vi "Klinger Goto.vi"(0 "Axe":u8(ring) items=["W", "X", "Y", "Z"], 1 "Suivi":T1={"CorrectPos"=TRUE, "Nb Essais Max"=5, "Erreur de suivi max"=1.0}, 2 "Moving Ref":refnum<vi>, 5 "Relatif":bool caption="Relatif/Absolu\n(Absolu)", 7 "UnitDem":u8(ring)=2 caption="Unités" items=["Pas", "mm", "ps"], 9 "PosDem":dbl=1.0 caption="Allez à" min=-7999999.9 max=7999999.9 step=0.1 format="%#_8f", 11 "error in":errorcluster, 12 "Position Ref":refnum<vi>) -> (3 "Moving":bool caption="Déplacement\nen cours", 4 "PLimit":bool caption="Limite +", 6 "NLimit":bool caption="Limite -", 8 "Pos Init":dbl caption="Position Initiale", 10 "Position":dbl format="%#.1f", 13 "PosErreur":dbl caption="Erreur de\nPositionnement", 14 "Indcomm":string caption="Indicateur de commande", 15 "error out":errorcluster)   [LabVIEW 2010]
doc: "Ce VI envoie une commande de déplacement au controlleur Klinger MC4. \n\nAxe : Sélectionner l'axe sur lequel effectuer le déplacement\n\nAllez à :En mode de déplacement absolu, entrer la position de destination en pas. En mode de déplacement relatif, entrer le nombre de pas à effectuer. Le signe indique la direcetion de déplacement. Valeur accepter :-7 999 999,9 à 7 999 999,9\n\nRelatif/Absolu : Choisi le type de déplacementà effectuer. En mode absolu, le déplacement est effectué par rapport à une position de référence prédéfini. En mode relatif, le déplacement est effectué par rapport à la position actuelle.\n\nLimite + : Indique l'atteinte de l'interrupeur de fin de course positif\n\nLimite - : Indique l'atteinte de l'interrupeur de fin de course négatif\n\nPosition: Indique la position finale"
uses:
  <vilib>/Utility/error.llb/DialogType.ctl
  Programmes LabView/Réflectivité Différentielle/Params Globals.vi
  <userlib>/Klinger/Klinger Lib.llb/Klinger ConvUnitSgl.vi
panel:
  out "NbEssais":i32
  out "Message D'erreur":string
  out "Erreur":bool
  # "Relatif"
  # "Absolu"
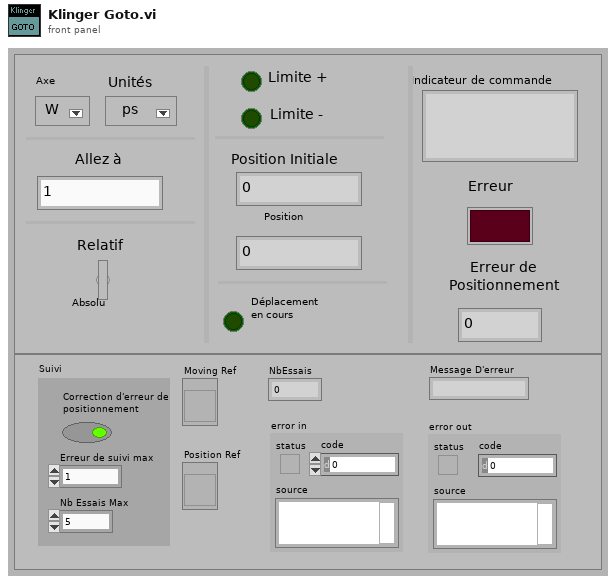
[diagram p1: front panel]
types:
  T1 = cluster{"CorrectPos":bool, "Nb Essais Max":i32, "Erreur de suivi max":dbl}
  T2 = enum16{"Dem Pos Init", "Lire Pos Init", "Envoie Comm", "Dem Statut", "Lire Statut", "Attend RQS", "Erreur GPIB", "Dépl incomp", "Dépl comp"}
  T3 = typedef "DialogType.ctl" = u16
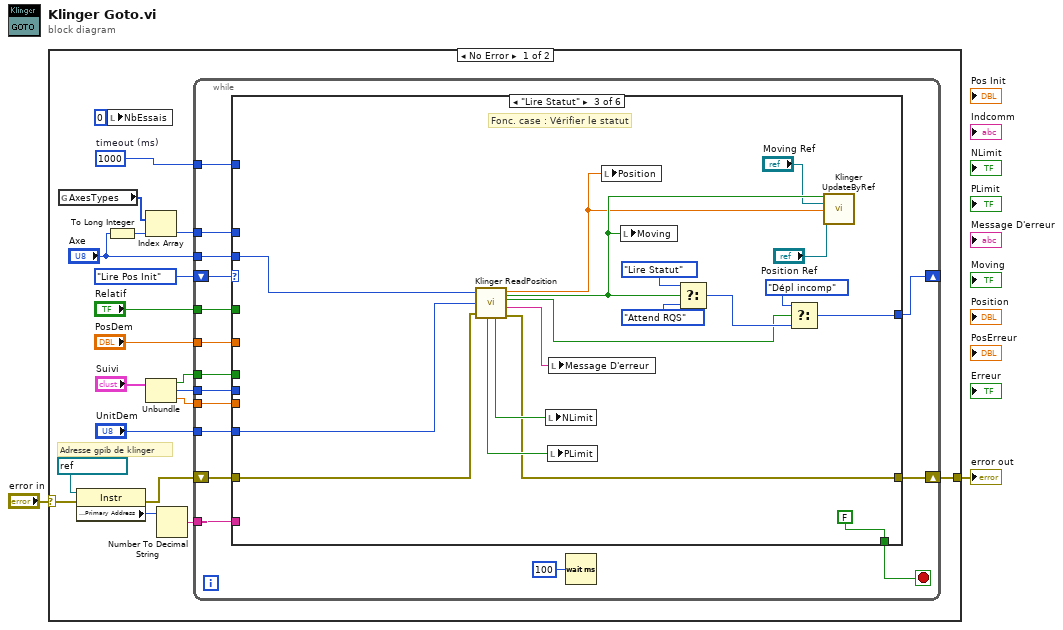
[diagram p0: block diagram]
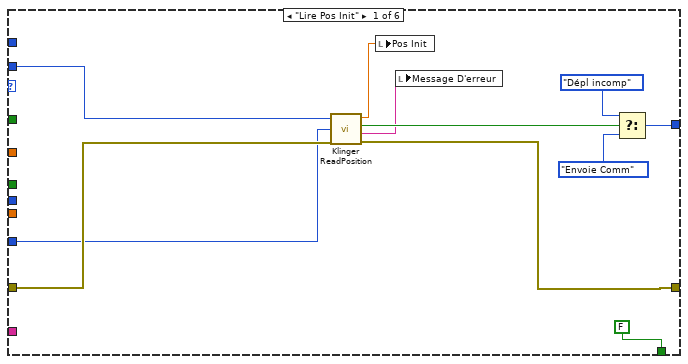
[diagram p2: hidden frame]
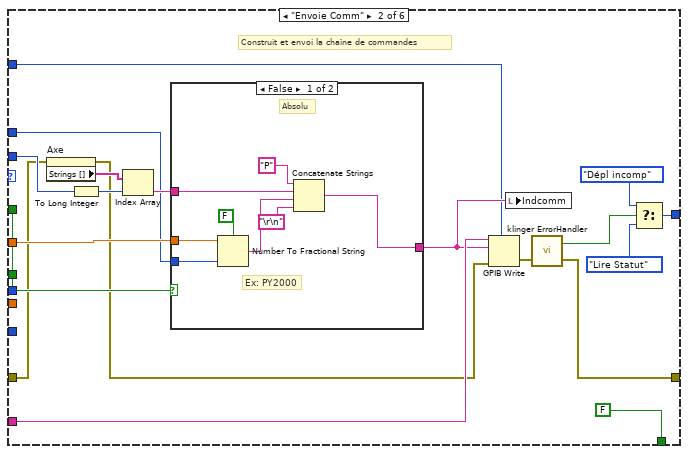
[diagram p3: hidden frame]
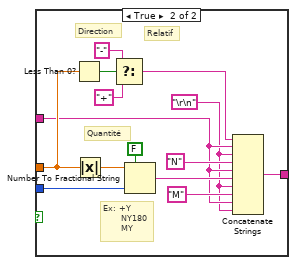
[diagram p4: hidden frame]
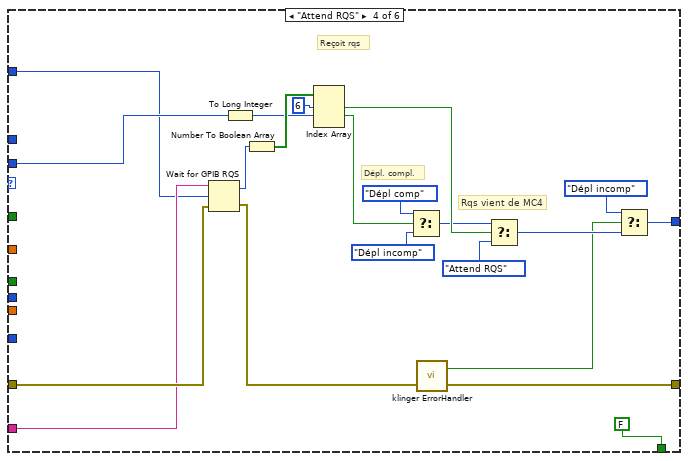
[diagram p5: hidden frame]
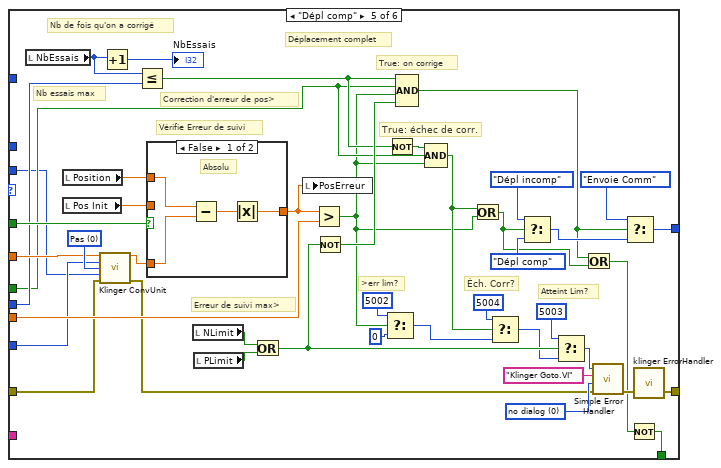
[diagram p6: hidden frame]
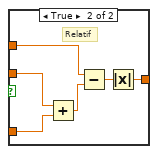
[diagram p7: hidden frame]
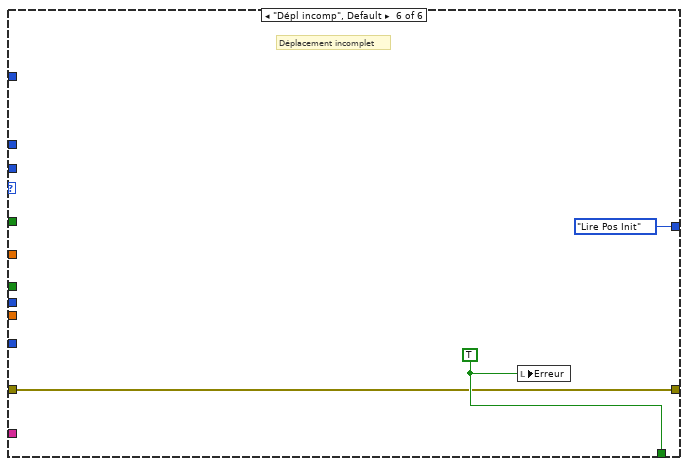
[diagram p8: hidden frame]
diagram:
  n1 = case shown="No Error" "error in" {
    selector: "error in" -> [w15 w187]
    tunnel: [w20 w187] -> w2
    frame No Error {
      w12 = 1000  # timeout (ms)
      # "Adresse gpib de klinger"
      n2 = global read "Params Globals.vi" "AxesTypes"() -> (w3:enum16{"UE30", "UE72"}[])
      n3 = property class="Instr"(reference=refnum<visa-resource-name> "KLINGER", error in=w15) -> (error out=w14:errorcluster, "GPIB Settings:Primary Address"=w18:u16)  [unwired: 1 out]
      n4 = To Long Integer(number="Axe") -> (32bit integer=w6:i32)
      n5 = local write "NbEssais"(0 ("Numeric")) -> ()
      n6 = Index Array(array=w3, index=w6) -> (element=w4:enum16{"UE30", "UE72"})
      n7 = Unbundle("Suivi") -> ("CorrectPos"=w8:bool, "Nb Essais Max"=w9:i32, "Erreur de suivi max"=w7:dbl)
      n8 = Number To Decimal String(number=w18) -> (decimal integer string=w16:string)  [unwired: 1 in]
      n9 = while {
        shift-right: [w37] -> w20
        shift-left: w14 -> [w36]
        tunnel: "Axe" -> [w35]
        tunnel: "PosDem" -> [w34]
        tunnel: "Relatif" -> [w33]
        tunnel: w12 -> [w32]
        shift-right: [w29] -> _
        shift-left: T2."Lire Pos Init" ("f") -> [w30]
        tunnel: w7 -> [w28]
        tunnel: w16 -> [w27]
        tunnel: "UnitDem" -> [w26]
        tunnel: w9 -> [w25]
        tunnel: w8 -> [w24]
        tunnel: w4 -> [w23]
        stop <- w38 stop-if-true
        n10 = case shown="\"Lire Statut\"" w30 {
          tunnel: [FALSE FALSE FALSE FALSE w166 w185] -> w38
          tunnel: [w45 w56 w95 w110 w163 w184] -> w37
          tunnel: w36 -> [w42 w52 w100 w129 w132 w184]
          tunnel: w35 -> [w41 w65 w91 w127 w133 _]
          tunnel: w34 -> [_ w54 _ _ w150 _]
          tunnel: w33 -> [_ w63 _ _ w173 _]
          tunnel: w27 -> [_ w62 _ w128 _ _]
          tunnel: w32 -> [_ w53 _ w118 _ _]
          tunnel: [w46 w59 w105 w113 w151 T2."Lire Pos Init" ("f")] -> w29
          tunnel: w28 -> [_ _ _ _ w172 _]
          tunnel: w26 -> [w39 _ w92 _ w149 _]
          tunnel: w25 -> [_ _ _ _ w135 _]
          tunnel: w24 -> [_ _ _ _ w134 _]
          tunnel: w23 -> [_ w50 _ _ _ _]
          frame "Lire Pos Init" {
            n11 = call <userlib>:"Klinger ReadPosition.vi"("Axe"=w41, "UnitDem"=w39, "error in"=w42) -> ("Position"=w40:dbl, "Statut"=w44:bool, "Cont Error"=w43:string, "error out"=w45:errorcluster)  [unwired: 1 in, 3 out]
            n12 = local write "Pos Init"(w40) -> ()
            n13 = local write "Message D'erreur"(w43) -> ()
            n14 = Select(t=T2."Dépl incomp", s=w44, f=T2."Envoie Comm") -> (s? t:f=w46:T2)
          }
          frame "Envoie Comm" {
            # "Construit et envoi la chaîne de commandes"
            n15 = property on="Axe" class="Ring (strict)"(error in=w52) -> (error out=w51:errorcluster, "Strings []"=w68:string[])  [unwired: 1 in, 1 out]
            n16 = To Long Integer(number=w65) -> (32bit integer=w64:i32)
            n17 = Index Array(array=w68, index=w64) -> (element=w67:string)
            n18 = case shown="False" w63 {
              tunnel: w54 -> [w76 w88]
              tunnel: w67 -> [w73 w80]
              tunnel: [w71 w78] -> w58
              tunnel: w50 -> [w69 w77]
              frame False {
                # "Ex: PY2000"
                # "Absolu"
                n19 = Number To Fractional String(use system decimal point (T)=FALSE, number=w76, precision (6)=w69) -> (F-format string=w75:string)  [unwired: 1 in]
                n20 = Concatenate Strings("P", w73, w75, "\r\n") -> (w71:string)
              }
              frame True {
                w79 = "\r\n"
                # "Quantité"
                # "Direction"
                # "Ex: +Y\n      NY180\n      MY"
                # "Relatif"
                n21 = Less Than 0?(x=w88) -> (x < 0?=w87:bool)
                n22 = Absolute Value(x=w88) -> (abs(x)=w90:dbl)
                n23 = Select(t="-", s=w87, f="+") -> (s? t:f=w84:string)
                n24 = Number To Fractional String(use system decimal point (T)=FALSE, number=w90, precision (6)=w77) -> (F-format string=w82:string)  [unwired: 1 in]
                n25 = Concatenate Strings(w84, w80, w79, "N", w80, w82, w79, "M", w80, w79) -> (w78:string)
              }
            }
            n26 = GPIB Write(0:w62, 1:w58, 3:w51, 4:w53) -> (6:w57:errorcluster)  [unwired: 1 in, 1 out]
            n27 = local write "Indcomm"(w58) -> ()
            n28 = call <userlib>:"klinger ErrorHandler.vi"("error in (no error)"=w57) -> ("error out"=w56:errorcluster, "Erreur"=w55:bool)  [unwired: 1 in]
            n29 = Select(t=T2."Dépl incomp", s=w55, f=T2."Lire Statut") -> (s? t:f=w59:T2)
          }
          frame "Lire Statut" {
            # "Fonc. case : Vérifier le statut"
            n30 = call <userlib>:"Klinger ReadPosition.vi"("Axe"=w91, "UnitDem"=w92, "error in"=w100) -> ("PLimit"=w99:bool, "Moving"=w96:bool, "Position"=w94:dbl, "Statut"=w101:bool, "NLimit"=w98:bool, "Cont Error"=w97:string, "error out"=w95:errorcluster)  [unwired: 1 in]
            n31 = local write "NLimit"(w98) -> ()
            n32 = local write "PLimit"(w99) -> ()
            n33 = local write "Message D'erreur"(w97) -> ()
            n34 = local write "Position"(w94) -> ()
            n35 = local write "Moving"(w96) -> ()
            n36 = Select(t=T2."Lire Statut", s=w96, f=T2."Attend RQS") -> (s? t:f=w103:T2)
            n37 = Select(t=T2."Dépl incomp", s=w101, f=w103) -> (s? t:f=w105:T2)
            n38 = call <userlib>:"Klinger UpdateByRef.vi"("Moving?"=w96, "Moving Ref"="Moving Ref", "Position"=w94, "Position Ref"="Position Ref") -> ()  [unwired: 11 in, 1 out]
          }
          frame "Attend RQS" {
            # "Dépl. compl."
            # "Rqs vient de MC4"
            # "Reçoit rqs"
            n39 = Wait for GPIB RQS(2:w129, 3:w118, 4:w128) -> (0:w117:errorcluster, 1:w125:i16)
            n40 = To Long Integer(number=w127) -> (32bit integer=w121:i32)
            n41 = Number To Boolean Array(number=w125) -> (Boolean array=w126:bool[])
            n42 = Index Array(array=w126, index #1=6 ("index"), index #2=w121) -> (element #1=w123:bool, element #2=w120:bool)  [unwired: 1 in, 1 out]
            n43 = Select(t=T2."Dépl comp", s=w120, f=T2."Dépl incomp") -> (s? t:f=w119:T2)
            n44 = call <userlib>:"klinger ErrorHandler.vi"("error in (no error)"=w117) -> ("error out"=w110:errorcluster, "Erreur"=w109:bool)  [unwired: 1 in]
            n45 = Select(t=w119, s=w123, f=T2."Attend RQS") -> (s? t:f=w112:T2)
            n46 = Select(t=T2."Dépl incomp", s=w109, f=w112) -> (s? t:f=w113:T2)
          }
          frame "Dépl comp" {
            w160 = u8 0 items=["Pas", "mm", "ps"] ("UnitAct")
            w168 = T3 0 items=["no dialog", "OK message", "continue or stop message", "OK message + warnings", "continue/stop + warnings"] ("type of dialog (OK msg:1)")
            # "Nb essais max"
            # "Correction d'erreur de pos>"
            # "Erreur de suivi max>"
            # ">err lim?"
            # "Éch. Corr?"
            # "Atteint Lim?"
            # "Nb de fois qu'on a corrigé"
            # "True: échec de corr."
            # "True: on corrige"
            # "Vérifie Erreur de suivi"
            # "Déplacement complet"
            n47 = local read "NbEssais"() -> (w158:i32)
            n48 = local read "Position"() -> (w164:dbl)
            n49 = local read "Pos Init"() -> (w165:dbl)
            n50 = call-poly <userlib>:"Klinger ConvUnit.vi"("ParamAct"=w150, "UnitDem"=w149, "UnitAct"=w160, "Axe"=w133, "error in"=w132) -> ("ParamDem"=w159:dbl, "error out"=w131:errorcluster)  [unwired: 9 in]
            n51 = Increment(x=w158) -> (x+1=→"NbEssais":i32)
            n52 = Less Or Equal?(x=w158, y=w135) -> (x <= y?=w153:bool)
            n53 = case shown="False" w173 {
              tunnel: w165 -> [_ w182]
              tunnel: w159 -> [w176 w181]
              tunnel: [w175 w179] -> w157
              tunnel: w164 -> [w174 w178]
              frame False {
                # "Absolu"
                n54 = Subtract(x=w174, y=w176) -> (x-y=w177:dbl)
                n55 = Absolute Value(x=w177) -> (abs(x)=w175:dbl)
              }
              frame True {
                # "Relatif"
                n56 = Add(x=w182, y=w181) -> (x+y=w183:dbl)
                n57 = Subtract(x=w178, y=w183) -> (x-y=w180:dbl)
                n58 = Absolute Value(x=w180) -> (abs(x)=w179:dbl)
              }
            }
            n59 = local read "NLimit"() -> (w162:bool)
            n60 = local read "PLimit"() -> (w161:bool)
            n61 = Or(x=w162, y=w161) -> (x .or. y?=w146:bool)
            n62 = local write "PosErreur"(w157) -> ()
            n63 = Greater?(x=w157, y=w172) -> (0:w130:bool)
            n64 = Not(x=w146) -> (.not. x?=w155:bool)
            n65 = Select(t=5002 ("error code (no error:0)"), s=w130, f=0 ("error code (no error:0)")) -> (s? t:f=w142:i32)
            n66 = Not(x=w153) -> (.not. x?=w148:bool)
            n67 = Compound Arithmetic op=AND(w153, w134, w130, w155) -> (w138:bool)
            n68 = Compound Arithmetic op=AND(w148, w134, w130) -> (w143:bool)
            n69 = Or(x=w143, y=w130) -> (x .or. y?=w139:bool)
            n70 = Select(t=5004 ("error code (no error:0)"), s=w143, f=w142) -> (s? t:f=w140:i32)
            n71 = Select(t=T2."Dépl incomp", s=w139, f=T2."Dépl comp") -> (s? t:f=w152:T2)
            n72 = Select(t=5003, s=w146, f=w140) -> (s? t:f=w144:i32)
            n73 = Or(x=w138, y=w139) -> (x .or. y?=w137:bool)
            n74 = call <vilib>:"Simple Error Handler.vi"("error code (no error:0)"=w144, "error source (\" \")"="Klinger Goto.VI" ("error source (\" \")"), "type of dialog (OK msg:1)"=w168, "error in (no error)"=w131) -> ("error out"=w169:errorcluster)  [unwired: 1 in, 4 out]
            n75 = Select(t=T2."Envoie Comm", s=w138, f=w152) -> (s? t:f=w151:T2)
            n76 = Not(x=w137) -> (.not. x?=w166:bool)
            n77 = call <userlib>:"klinger ErrorHandler.vi"("error in (no error)"=w169) -> ("error out"=w163:errorcluster)  [unwired: 1 in, 1 out]
          }
          frame "Dépl incomp", Default {
            w185 = TRUE
            # "Déplacement incomplet"
            n78 = local write "Erreur"(w185) -> ()
          }
        }
        n79 = Wait (ms)(milliseconds to wait=u32 100) -> ()  [unwired: 1 out]
      }
    }
    frame Error {
    }
  }
  "error out" <- w2
